vi "ReadContent.vi"(8 "error in (no error)":errorcluster, 11 "object in":refnum<class "inspect_request Message.lvclass">) -> (0 "error out":errorcluster, 2 "content":string, 3 "object out":refnum<class "inspect_request Message.lvclass">)   [LabVIEW 2018, in "ClientMessaging.lvlib" / "inspect_request Message.lvclass"]
uses:
  inspect_request Message.lvclass
  d80d35bc-50b2-4502-8d07-469129d111cd.vi
  Base Classes/Request Message/Request Message.lvclass
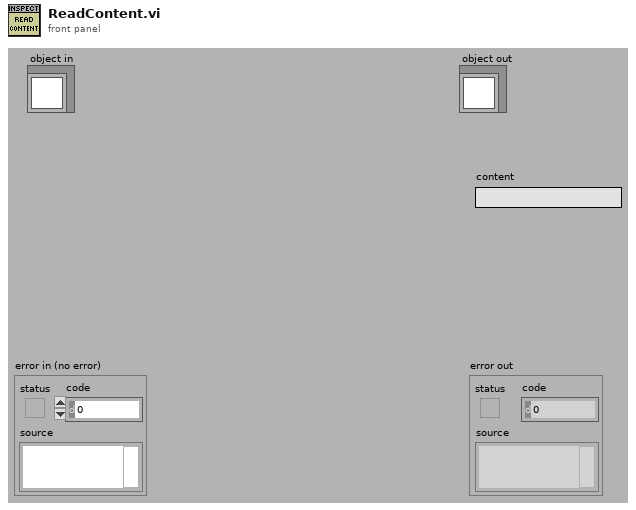
[diagram p1: front panel]
types:
  T1 = typedef "ClientMessaging.lvlib/inspect_request Message.lvclass/inspect content.ctl" = cluster{"code":string, "cursor_pos":u32, "detail_level":u8}
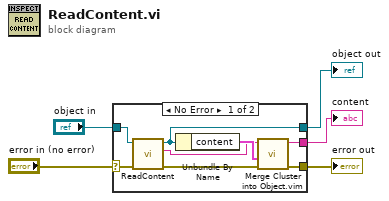
[diagram p0: block diagram]
diagram:
  n1 = case shown="No Error" "error in (no error)" {
    selector: "error in (no error)" -> [w7 w15]
    tunnel: [w6 w15] -> w3
    tunnel: [w11 w14] -> w1
    tunnel: "object in" -> [w13 w14]
    tunnel: [w8 _] -> w2
    frame No Error {
      n2 = call-parent "ReadContent.vi"("error in (no error)"=w7, "object in"=w13) -> ("error out"=w9:errorcluster, "content"=w10:string, "object out"=w11:refnum<class "inspect_request Message.lvclass">)  [unwired: 7 in]
      n3 = Unbundle By Name(w11) -> ("content"=w12:T1)
      n4 = call "Merge Cluster into Object.vim"("error in (no error)"=w9, "Any Cluster"=w12, "JSON"=w10) -> ("error out"=w6:errorcluster, "<JSON>"=w8:string)  [unwired: 6 in]
    }
    frame Error {
    }
  }
  "error out" <- w3
  "object out" <- w1
  "content" <- w2
